vi "Check Signal Direction.vi"(8 "error in (no error)":errorcluster, 11 "Module in":refnum<class "Module.lvclass">) -> (0 "error out":errorcluster, 3 "Module out":refnum<class "Module.lvclass">)   [LabVIEW 2025, in "Module.lvclass"]
doc: "Check the configuration for errors. Specifically make sure the signal IP direction matches the IO."
uses:
  Module.lvclass
  Module.lvclass/Module.ctl
  VI/VI/Error Codes.ctl
  Signal/Signal/Signal.lvclass/Signal.ctl
  Signal/Signal/Read Signal Type.vi
  Read Model Number.vi
  Read Name.vi
  Signal/Signal/Read IO Name.vi
  Signal/Signal/Read Signal Name.vi
  VI/VI/VI.lvclass
  Signal/Signal/Signal.lvclass
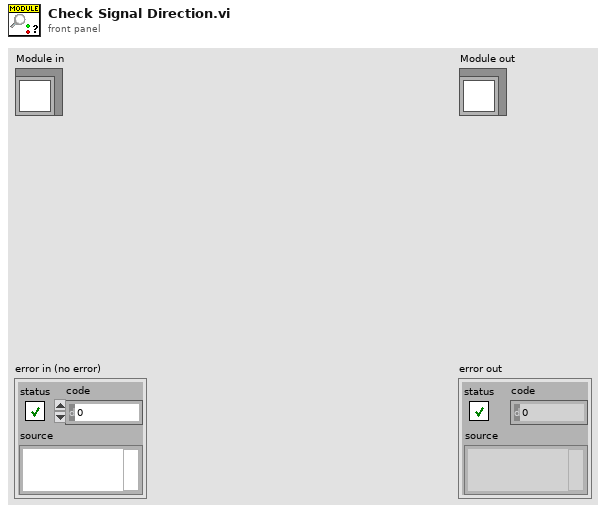
[diagram p1: front panel]
types:
  T1 = typedef "VI.lvclass/Error Codes.ctl" = enum16{"Signal Unsupported", "Module Unsupported", "Parameter Unsupported", "Signal Code Gen Error", "Module Code Gen Error", "Cleanup Code Error", "Signal Direction Mismatch", "Signal Type Mismatch", "Module Channel Number Mismatch", "Minimum Channels Mismatch"}
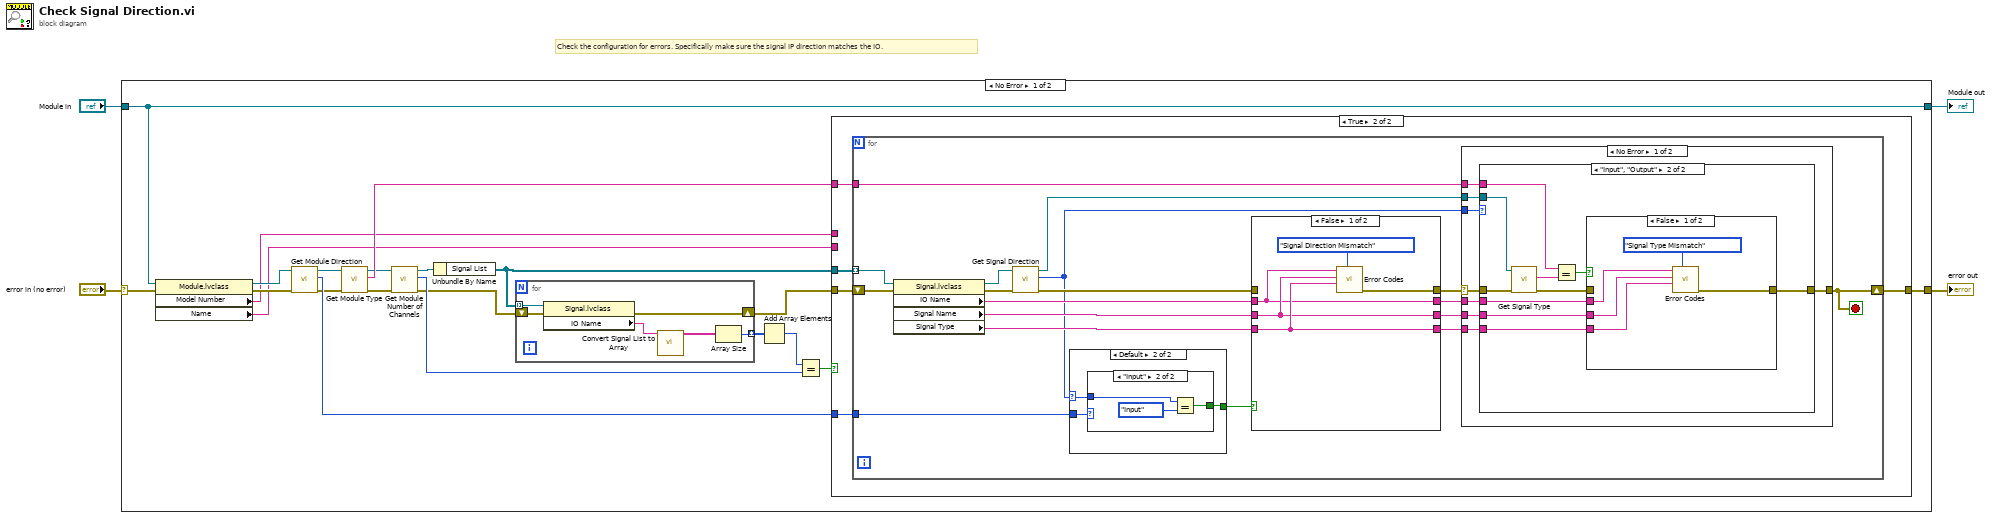
[diagram p0: block diagram]
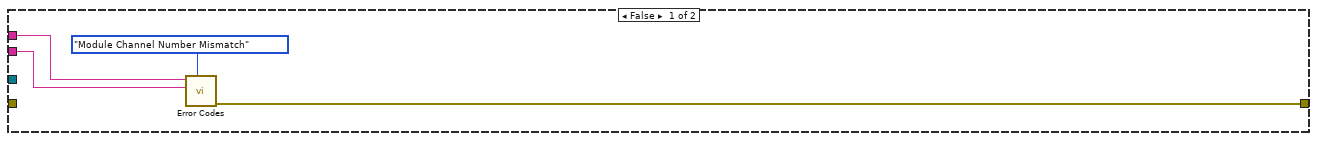
[diagram p2: hidden frame]
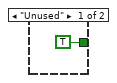
[diagram p7: hidden frame]
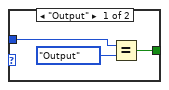
[diagram p8: hidden frame]
diagram:
  # "Check the configuration for errors. Specifically make sure the signal IP direction matches the IO."
  n1 = case shown="No Error" "error in (no error)" {
    selector: "error in (no error)" -> [w15 w105]
    tunnel: [w25 w105] -> w3
    tunnel: [w13 w104] -> w1
    tunnel: "Module in" -> [w13 w104]
    frame No Error {
      n2 = property class="Module.lvclass"(reference=w13, error in=w15) -> (reference out=w12:refnum<class "Module.lvclass">, error out=w14:errorcluster, "Model Number"=w11:string, "Name"=w10:string)
      n3 = call "Get Module Direction.vi"("error in (no error)"=w14, "Module in"=w12) -> ("error out"=w23:errorcluster, "Direction"=w24:enum16{"Input", "Output"}, "Module out"=w22:refnum<class "Module.lvclass">)  [unwired: 7 in]
      n4 = call "Get Module Type.vi"("error in (no error)"=w23, "Module in"=w22) -> ("error out"=w20:errorcluster, "Type"=w21:string, "Module out"=w19:refnum<class "Module.lvclass">)  [unwired: 7 in]
      n5 = call "Get Module Number of Channels.vi"("error in (no error)"=w20, "Module in"=w19) -> ("error out"=w8:errorcluster, "# of Channels"=w17:i32, "Module out"=w18:refnum<class "Module.lvclass">)  [unwired: 7 in]
      n6 = Unbundle By Name(w18) -> ("Signal List"=w9:refnum<class "Signal.lvclass">[])
      n7 = for {
        tunnel: w9 -> [w31] mode=indexing
        shift-right: [w29] -> w7
        shift-left: w8 -> [w30]
        tunnel: [w28] -> w6 mode=indexing
        n8 = property class="Signal.lvclass"(reference=w31, error in=w30) -> (error out=w29:errorcluster, "IO Name"=w27:string)  [unwired: 1 out]
        n9 = call "Convert Signal List to Array.vi"("Signal List"=w27) -> ("Signal List"=w26:string[])  [unwired: 10 in]
        n10 = Array Size(array=w26) -> (size(s)=w28:i32)
      }
      n11 = Add Array Elements(numeric array=w6) -> (sum=w5:i32)
      n12 = Equal?(x=w5, y=w17) -> (x = y?=w16:bool)
      n13 = case shown="True" w16 {
        tunnel: [w32 w40] -> w25
        tunnel: w24 -> [_ w39]
        tunnel: w21 -> [_ w38]
        tunnel: w9 -> [_ w37]
        tunnel: w7 -> [_ w36]
        tunnel: w11 -> [w34 _]
        tunnel: w10 -> [w33 _]
        frame False {
          n14 = call "Error Codes.vi"("Error"=Error_Codes."Module Channel Number Mismatch", "Module/Signal Name"=w33, "Module/Signal Resource"=w34) -> ("error out"=w32:errorcluster)  [unwired: 8 in]
        }
        frame True {
          n15 = for {
            tunnel: w37 -> [w56] mode=indexing
            shift-right: [w50] -> w40
            shift-left: w36 -> [w57]
            tunnel: w39 -> [w58]
            tunnel: w38 -> [w41]
            stop <- w50 stop-if-true
            n16 = property class="Signal.lvclass"(reference=w56, error in=w57) -> (reference out=w51:refnum<class "Signal.lvclass">, error out=w55:errorcluster, "IO Name"=w54:string, "Signal Name"=w53:string, "Signal Type"=w52:string)
            n17 = call "Get Signal Direction.vi"("error in (no error)"=w55, "IO Class in"=w51) -> ("error out"=w45:errorcluster, "Direction"=w43:enum16{"Input", "Output", "Unused"}, "IO Class out"=w44:refnum<class "Signal.lvclass">)  [unwired: 7 in]
            n18 = case shown="Default" w43 {
              selector: w43 -> [_ w96]
              tunnel: w58 -> [_ w97]
              tunnel: [TRUE w95] -> w46
              frame "Unused" {
              }
              frame Default {
                n19 = case shown="\"Input\"" w97 {
                  tunnel: w96 -> [w100 w103]
                  tunnel: [w98 w101] -> w95
                  frame "Output" {
                    n20 = Equal?(x=w100, y=enum16{"Input", "Output", "Unused"}."Output" ("Direction")) -> (x = y?=w98:bool)
                  }
                  frame "Input" {
                    n21 = Equal?(x=w103, y=enum16{"Input", "Output", "Unused"}."Input" ("Direction")) -> (x = y?=w101:bool)
                  }
                }
              }
            }
            n22 = case shown="False" w46 {
              tunnel: w45 -> [_ w93]
              tunnel: [w89 w93] -> w42
              tunnel: w54 -> [w85 w90]
              tunnel: w53 -> [w86 w91]
              tunnel: w52 -> [w87 w92]
              tunnel: [w87 w92] -> w49
              tunnel: [w86 w91] -> w48
              tunnel: [w85 w90] -> w47
              frame False {
                n23 = call "Error Codes.vi"("Error"=Error_Codes."Signal Direction Mismatch", "Signal Type"=w87, "Module/Signal Name"=w86, "Module/Signal Resource"=w85) -> ("error out"=w89:errorcluster)  [unwired: 7 in]
              }
              frame True {
              }
            }
            n24 = case shown="No Error" w42 {
              selector: w42 -> [w60 w84]
              tunnel: [w66 w84] -> w50
              tunnel: w49 -> [w65 _]
              tunnel: w48 -> [w64 _]
              tunnel: w47 -> [w63 _]
              tunnel: w44 -> [w62 _]
              tunnel: w43 -> [w61 _]
              tunnel: w41 -> [w59 _]
              frame No Error {
                n25 = case shown="\"Input\", \"Output\"" w61 {
                  tunnel: w60 -> [w67 w74]
                  tunnel: [w67 w73] -> w66
                  tunnel: w65 -> [_ w72]
                  tunnel: w64 -> [_ w71]
                  tunnel: w63 -> [_ w70]
                  tunnel: w62 -> [_ w69]
                  tunnel: w59 -> [_ w68]
                  frame "Unused" {
                  }
                  frame "Input", "Output" {
                    n26 = call "Get Signal Type.vi"("error in (no error)"=w74, "IO Class in"=w69) -> ("error out"=w76:errorcluster, "Type"=w77:string)  [unwired: 7 in, 1 out]
                    n27 = Equal?(x=w68, y=w77) -> (x = y?=w75:bool)
                    n28 = case shown="False" w75 {
                      tunnel: w76 -> [_ w83]
                      tunnel: [w82 w83] -> w73
                      tunnel: w70 -> [w78 _]
                      tunnel: w71 -> [w79 _]
                      tunnel: w72 -> [w80 _]
                      frame False {
                        n29 = call "Error Codes.vi"("Error"=Error_Codes."Signal Type Mismatch", "Signal Type"=w80, "Module/Signal Name"=w79, "Module/Signal Resource"=w78) -> ("error out"=w82:errorcluster)  [unwired: 7 in]
                      }
                      frame True {
                      }
                    }
                  }
                }
              }
              frame Error {
              }
            }
          }
        }
      }
    }
    frame Error {
    }
  }
  "error out" <- w3
  "Module out" <- w1
